vi "full stop XYZ.vi"(8 "error in (no error)":errorcluster, 11 "ASI stage":T1) -> (0 "error out":errorcluster)   [LabVIEW 2010]
uses:
  stage properties.ctl
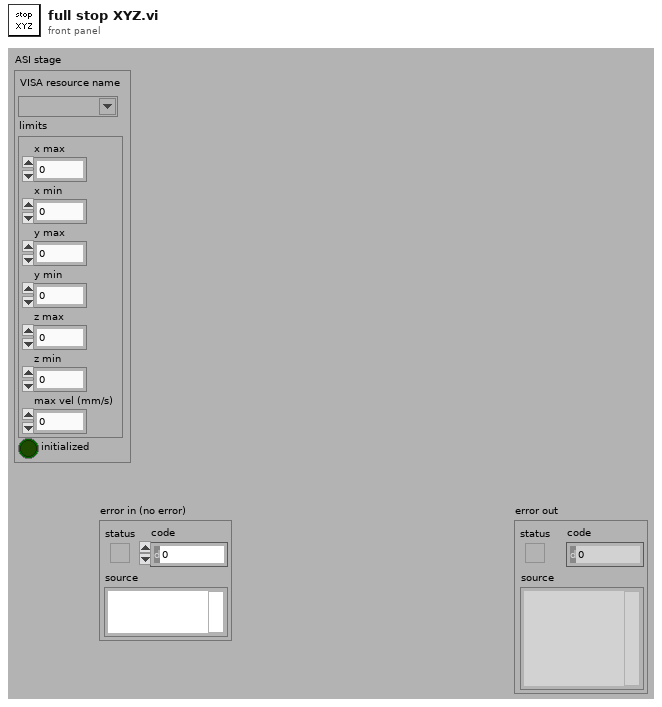
[diagram p1: front panel]
types:
  T1 = typedef "stage properties.ctl" = cluster{"VISA resource name":refnum<visa-resource-name>, "limits":cluster{"x max":dbl, "x min":dbl, "y max":dbl, "y min":dbl, "z max":dbl, "z min":dbl, "max vel (mm/s)":dbl}, "initialized":bool}
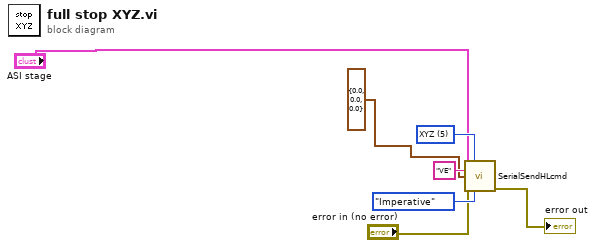
[diagram p0: block diagram]
diagram:
  w7 = u16 5 items=["No axis", "X", "Y", "Z", "XY", "XYZ"] ("Axis configuration")
  n1 = call "SerialSendHLcmd.vi"("ASI stage"="ASI stage", "Axis configuration"=w7, "Command"="VE", "data in"=cluster{"X in":dbl, "Y in":dbl, "Z in":dbl} {"X in"=0.0, "Y in"=0.0, "Z in"=0.0}, "error in (no error)"="error in (no error)", "Command type"=enum16{"Query", "Where", "Imperative", "DU Y"}."Imperative") -> ("error out"=→"error out":errorcluster)  [unwired: 7 in, 2 out]
